vi "Create Pattern Script(ChipID).vi"(8 "error in (no error)":errorcluster, 11 "ChipID":u8) -> (0 "error out":errorcluster, 3 "Script out":string)   [LabVIEW 2018, in "BML_Frame_Root.lvclass"]
uses:
  BML_Frame_Root.lvclass
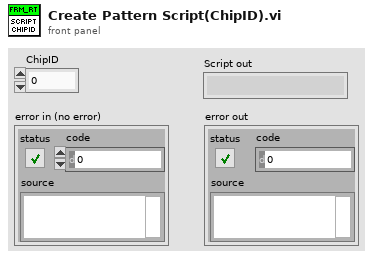
[diagram p1: front panel]
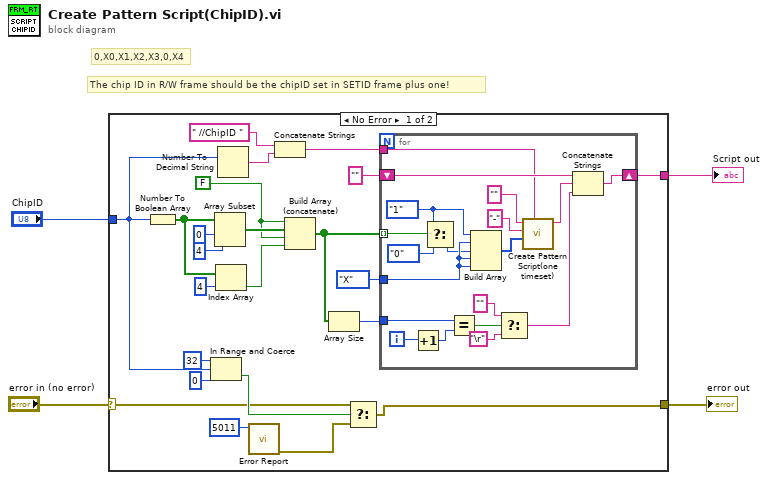
[diagram p0: block diagram]
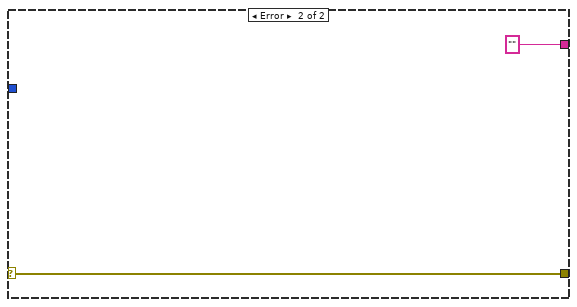
[diagram p2: hidden frame]
diagram:
  # "The chip ID in R/W frame should be the chipID set in SETID frame plus one!"
  # "0,X0,X1,X2,X3,0,X4"
  n1 = case shown="No Error" "error in (no error)" {
    selector: "error in (no error)" -> [w12 w47]
    tunnel: "ChipID" -> [w5 _]
    tunnel: [w19 ""] -> w2
    tunnel: [w10 w47] -> w1
    frame No Error {
      w21 = FALSE
      n2 = Number To Boolean Array(number=w5) -> (Boolean array=w25:bool[])
      n3 = In Range and Coerce(upper limit=u8 32, x=w5, lower limit=u8 0) -> (In Range?=w13:bool)  [unwired: 1 out]
      n4 = Array Subset(array=w25, index=0, length=4) -> (w23:bool[])
      n5 = Index Array(array=w25, index=4) -> (element=w22:bool)
      n6 = Number To Decimal String(number=w5) -> (decimal integer string=w7:string)  [unwired: 1 in]
      n7 = call "Error Report.vi"("Error Code"=i16 5011) -> ("error out"=w11:errorcluster)  [unwired: 10 in]
      n8 = Concatenate Strings(" //ChipID " ("Notes"), w7) -> (w6:string)
      n9 = Build Array (concatenate)(w21, w23, w21, w22) -> (w18:bool[])
      n10 = Array Size(array=w18) -> (size(s)=w17:i32)
      n11 = Select(t=w12, s=w13, f=w11) -> (s? t:f=w10:errorcluster)
      n12 = for {
        tunnel: w18 -> [w46] mode=indexing
        shift-right: [w44] -> w19
        shift-left: "" -> [w43]
        tunnel: w17 -> [w40]
        tunnel: enum16{"0", "1", "L", "H", "X", "V", "D", "M"}."X" ("PinState") -> [w31]
        tunnel: w6 -> [w28]
        i -> [w42]
        w30 = enum16{"0", "1", "L", "H", "X", "V", "D", "M"}."1" ("PinState")
        n13 = Increment(x=w42) -> (x+1=w41:i32)
        n14 = Select(t=w30, s=w46, f=enum16{"0", "1", "L", "H", "X", "V", "D", "M"}."0" ("PinState")) -> (s? t:f=w29:enum16{"0", "1", "L", "H", "X", "V", "D", "M"})
        n15 = Equal?(x=w40, y=w41) -> (x = y?=w39:bool)
        n16 = Build Array(w30, w31, w29, w31, w31) -> (w35:enum16{"0", "1", "L", "H", "X", "V", "D", "M"}[])
        n17 = Select(t="", s=w39, f="\r") -> (s? t:f=w36:string)
        n18 = call "Create Pattern Script(one timeset).vi"("Notes"=w28, "PinState"=w35, "timeset name"="-", "opcode"="") -> ("string out"=w32:string)  [unwired: 7 in]
        n19 = Concatenate Strings(w43, w32, w36) -> (w44:string)
      }
    }
    frame Error {
    }
  }
  "Script out" <- w2
  "error out" <- w1
